vi "Do.vi"(8 "error in (no error)":errorcluster, 10 "Actor in":refnum<class "Actor.lvclass">, 11 "Register Disabled Undo Msg in":refnum<class "Register Disabled Undo Msg.lvclass">) -> (0 "error out":errorcluster, 2 "Actor out":refnum<class "Actor.lvclass">)   [LabVIEW 2020, in "Map Model.lvlib" / "Register Disabled Undo Msg.lvclass"]
doc: "(<B>Filename</B>: Actor Framework.lvlib:Message.lvclass:Do.vi)\n\nDefines what a message does when it is received by an actor. Generally, a message instructs an actor to invoke one of its methods.\n\nBy default, this method does nothing. A child class must override it to define behavior. Create a child class by using the Actor Framework Message Maker dialog box."
uses:
  Register Disabled Undo Msg.lvclass
  <vilib>/ActorFramework/Actor/Actor.lvclass
  Map Model/Map Model.lvclass
  C:/Program Files/National Instruments/LabVIEW 2020/vi.lib/ActorFramework/Actor/Actor.lvclass
panel:
  # "NOTICE -- YOU MUST LEAVE THIS NOTICE IN PLACE.\n\nCopyright (c) 2017, LIANG LIU Shawn.Liu.cn@gmail.com\nAll rights reserved.\n\nRedistribution and use in source and binary forms, with or without modification, are permitted provided that the following conditions are met:\n-Redistributions of source code must retain the above copyright notice, this list of conditions and the following disclaimer.\n-Redistributions in binary form must reproduce the above copyright notice, this list of conditions and the following disclaimer in the documentation and/or other materials provided with the distribution.\n-Neither the name of the eLp nor the names of its contributors may be used to endorse or promote products derived from this software without specific prior written permission.\n\nTHIS SOFTWARE IS PROVIDED BY THE COPYRIGHT HOLDERS AND CONTRIBUTORS \"AS IS\" AND ANY EXPRESS OR IMPLIED WARRANTIES, INCLUDING, BUT NOT LIMITED TO, THE IMPLIED WARRANTIES OF MERCHANTABILITY AND FITNESS FOR A PARTICULAR PURPOSE ARE DISCLAIMED. IN NO EVENT SHALL THE COPYRIGHT HOLDER OR CONTRIBUTORS BE LIABLE FOR ANY DIRECT, INDIRECT, INCIDENTAL, SPECIAL, EXEMPLARY, OR CONSEQUENTIAL DAMAGES (INCLUDING, BUT NOT LIMITED TO, PROCUREMENT OF SUBSTITUTE GOODS OR SERVICES; LOSS OF USE, DATA, OR PROFITS; OR BUSINESS INTERRUPTION) HOWEVER CAUSED AND ON ANY THEORY OF LIABILITY, WHETHER IN CONTRACT, STRICT LIABILITY, OR TORT (INCLUDING NEGLIGENCE OR OTHERWISE) ARISING IN ANY WAY OUT OF THE USE OF THIS SOFTWARE, EVEN IF ADVISED OF THE POSSIBILITY OF SUCH DAMAGE."
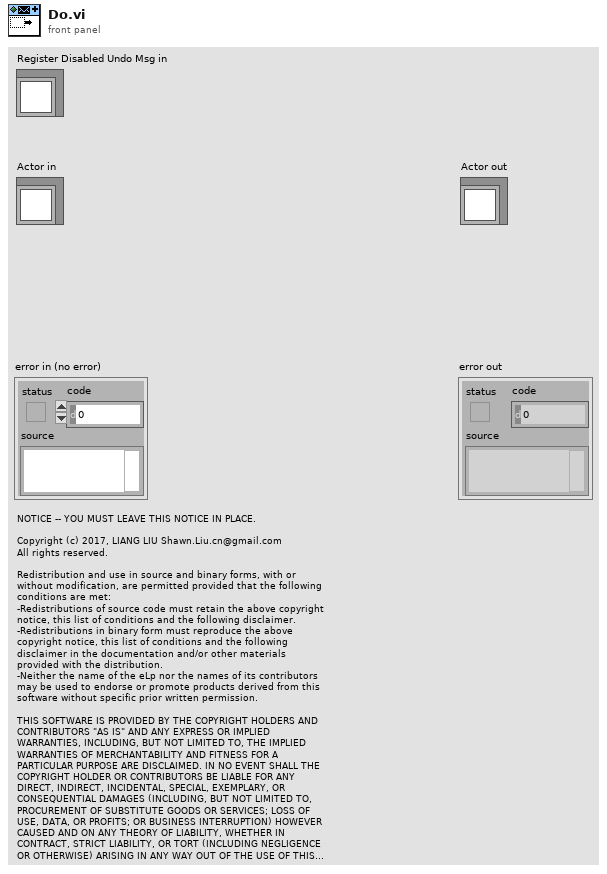
[diagram p1: front panel]
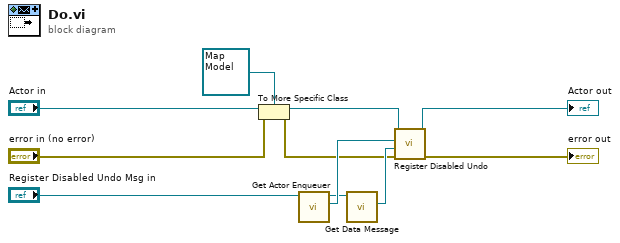
[diagram p0: block diagram]
diagram:
  n1 = To More Specific Class(target class=refnum<class "Map Model.lvclass"> refnum ("Map Model.lvlib:Map Model.lvclass"), reference="Actor in", error in="error in (no error)") -> (specific class reference=w2:refnum<class "Map Model.lvclass">, error out=w1:errorcluster)
  n2 = call-dynamic "Get Actor Enqueuer.vi"("Registration Message in"="Register Disabled Undo Msg in") -> ("Actor Enqueuer"=w7:refnum<class "Message Enqueuer.lvclass">, "Registration Message out"=w5:refnum<class "Register Disabled Undo Msg.lvclass">)  [unwired: 9 in]
  n3 = call-dynamic "Get Data Message.vi"("Registration Message in"=w5) -> ("Data Message"=w6:refnum<class "Data Message.lvclass">)  [unwired: 9 in, 1 out]
  n4 = call "Register Disabled Undo.vi"("error in (no error)"=w1, "Data Message"=w6, "View Enqueuer"=w7, "Map Model in"=w2) -> ("error out"=→"error out":errorcluster, "Map Model out"=→"Actor out":refnum<class "Map Model.lvclass">)  [unwired: 6 in]
